vi "Global.vi"() -> ()   [LabVIEW 2020]
panel:
  in  "Position":dbl
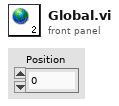
[diagram p1: front panel]
diagram:
